vi "五子棋_電腦對戰.vi"() -> ()   [LabVIEW 2019, in "五子棋.lvlib"]
uses:
  Status.ctl
  SetPiece.ctl
  <vilib>/numeric/Random Number (Range) U64.vi
  <vilib>/numeric/sub_Random U32.vi
panel:
  out "Info":string
  out "狀態":string
  out "黑子":T1[][](array[typedef])
  out "白子":T2[][](array[typedef])
  # "五子棋電腦對戰版"
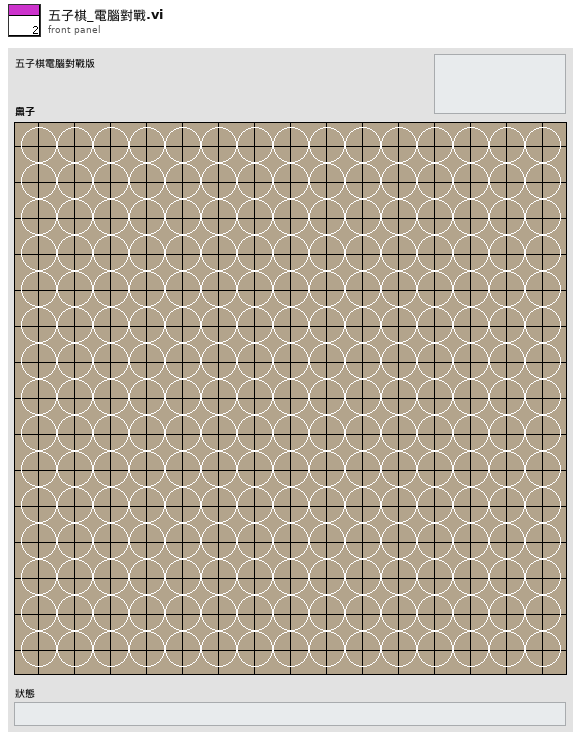
[diagram p1: front panel]
types:
  T1 = typedef "五子棋.lvlib/黑子.ctl" = bool
  T2 = typedef "五子棋.lvlib/白子.ctl" = bool
  T3 = typedef "五子棋.lvlib/SetPiece.ctl" = cluster{"Row":i32, "Col":i32, "Black?":bool}
  T4 = typedef "五子棋.lvlib/Status.ctl" = enum16{"Idle", "Initialize", "Set Piece", "Check Win", "Computer Play"}
  T5 = typedef "LVPositionTypeDef.ctl" = cluster{"Left":i32, "Top":i32}
  T6 = typedef "LVBoundsTypeDef.ctl" = cluster{"Width":u32, "Height":u32}
  T7 = cluster{"Number of Columns":u32, "Number of Rows":u32}
  T8 = typedef "Event 2-上課練習.lvlib/黑子.ctl" = bool
  T9 = typedef "Event 2-上課練習.lvlib/白子.ctl" = bool
  T10 = cluster{"Number of Columns":bool, "Number of Rows":bool}
  T11 = typedef "LVPoint32TypeDef.ctl" = cluster{"Horizontal":i32, "Vertical":i32}
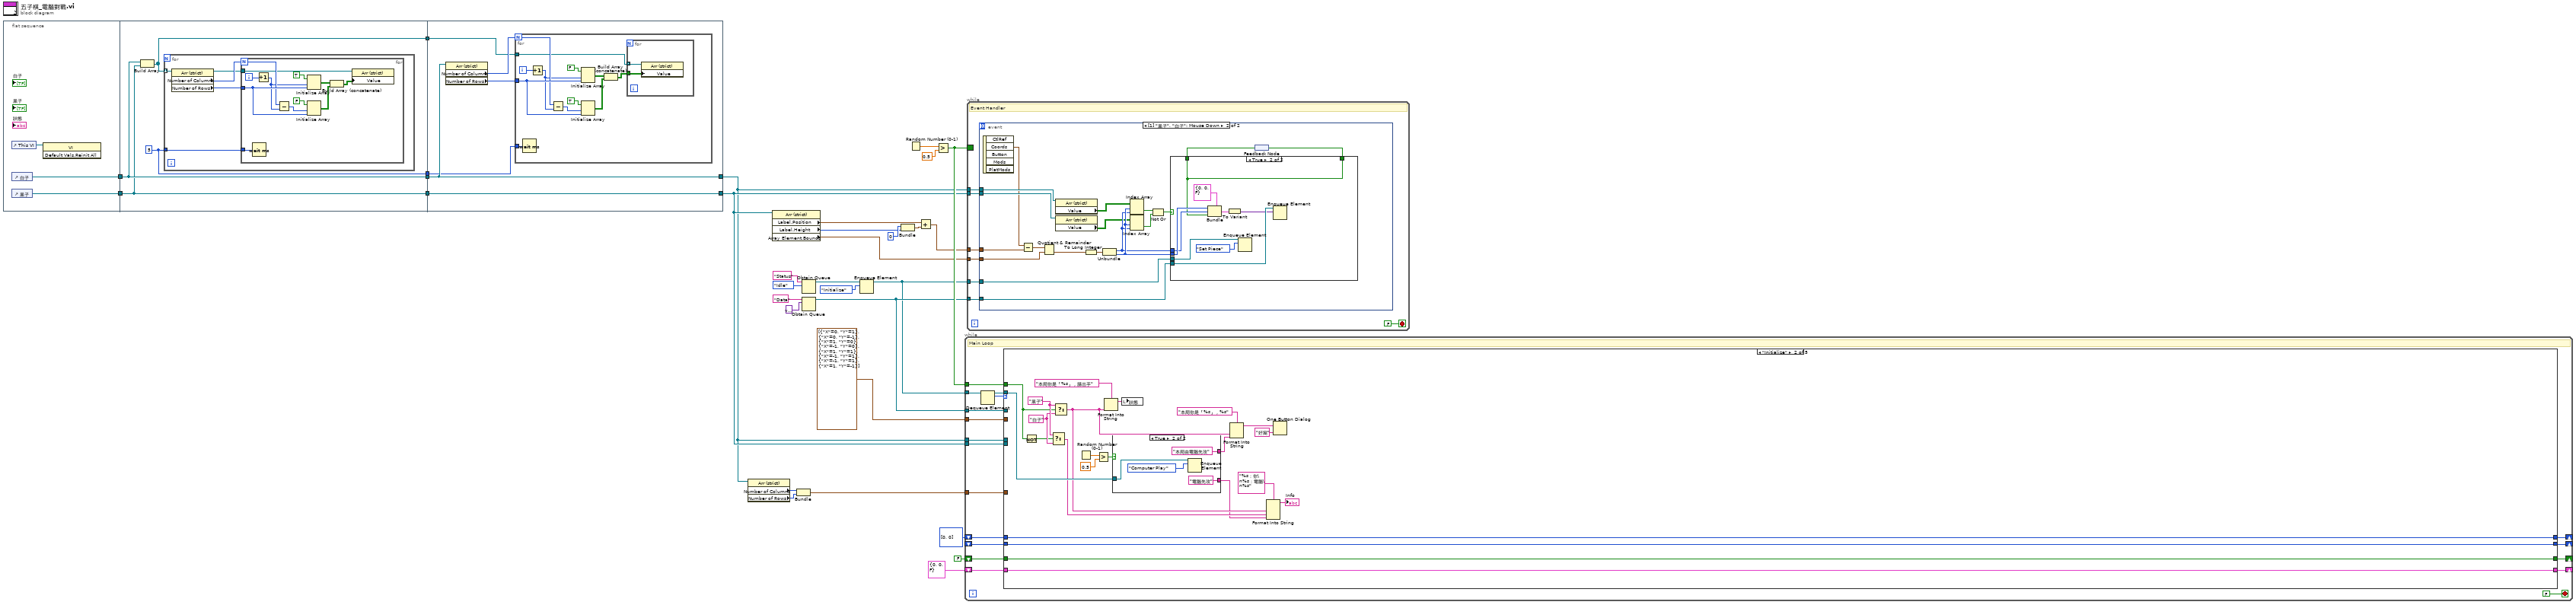
[diagram p0: block diagram]
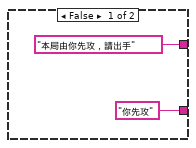
[diagram p3: hidden frame]
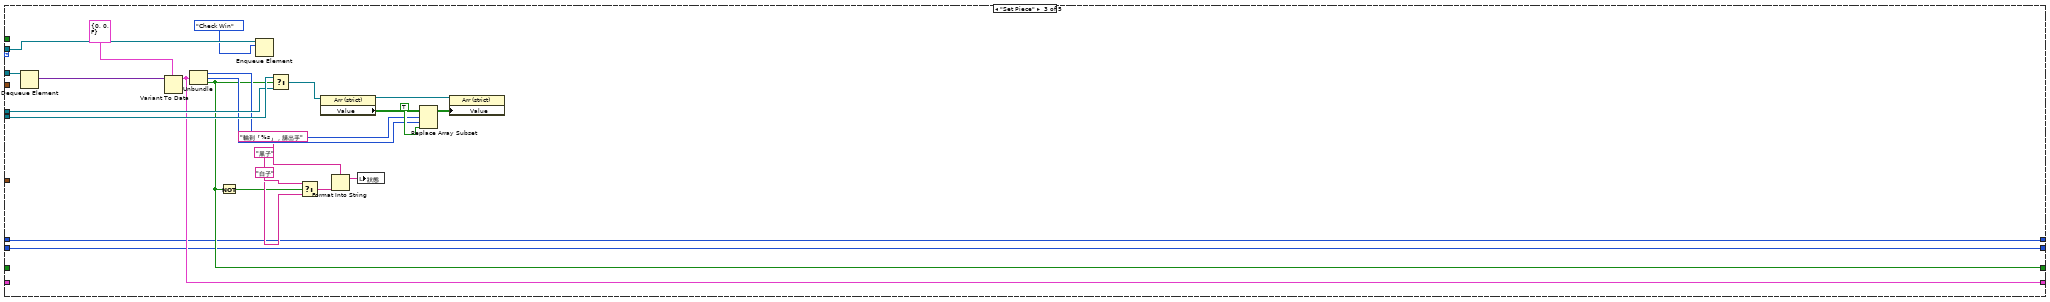
[diagram p4: hidden frame]
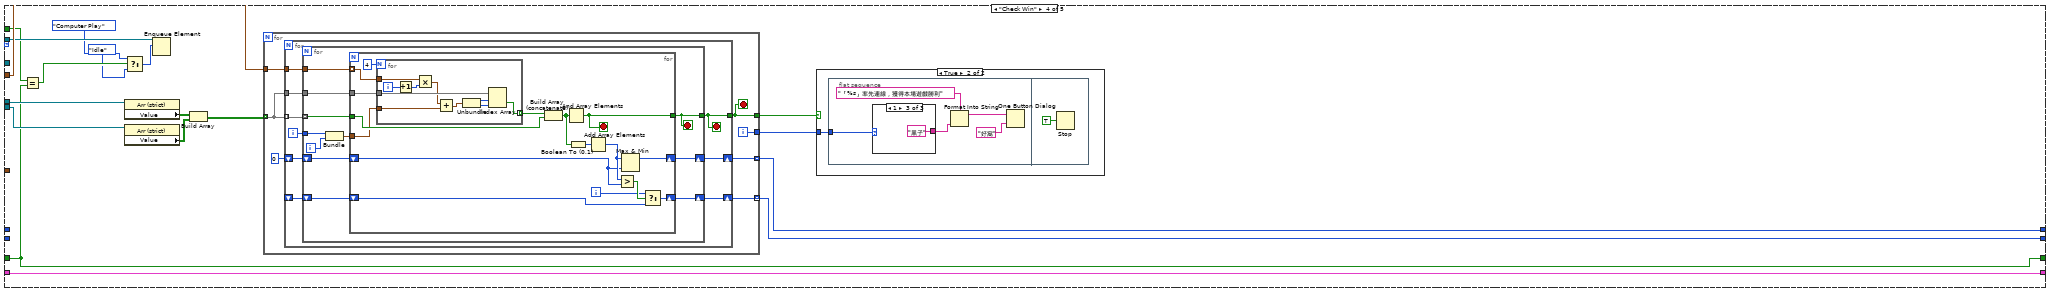
[diagram p5: hidden frame]
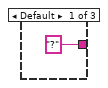
[diagram p7: hidden frame]
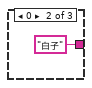
[diagram p8: hidden frame]
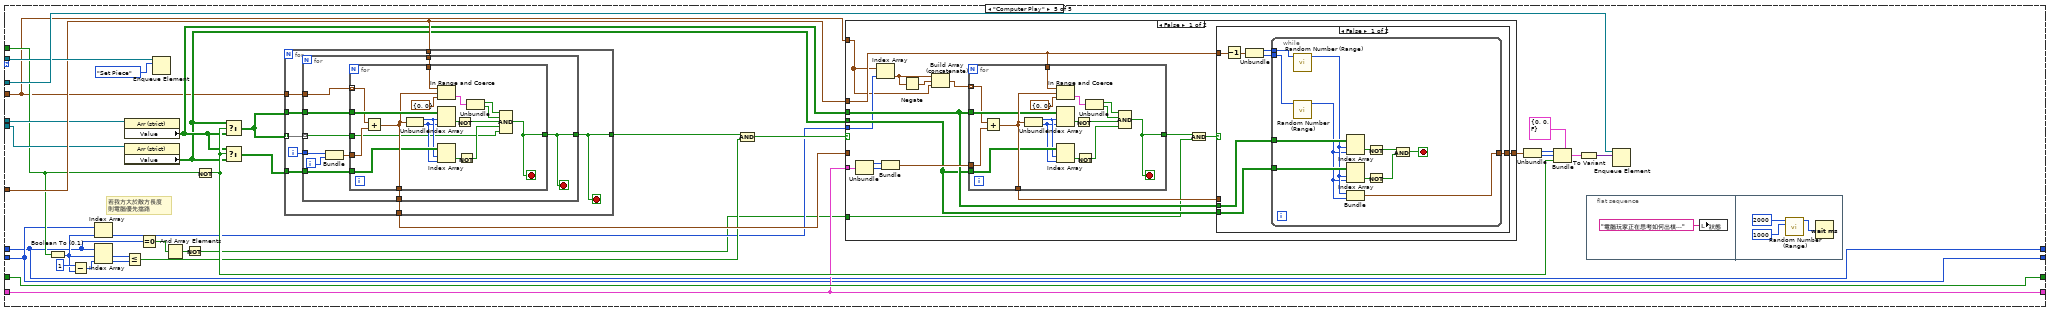
[diagram p9: hidden frame]
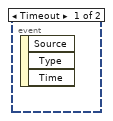
[diagram p12: hidden frame]
diagram:
  n1 = flat-sequence {
    tunnel: [w34] -> w15
    tunnel: [w33] -> w14
    tunnel: w15 -> [w38]
    tunnel: w14 -> [w39]
    tunnel: [w38] -> w13
    tunnel: [w39] -> w12
    tunnel: [w37] -> w11
    tunnel: [w36] -> w1
    tunnel: [w59] -> w8
    tunnel: [w62] -> w26
    tunnel: w13 -> [w62]
    tunnel: w12 -> [w59]
    tunnel: w11 -> [w58]
    tunnel: w1 -> [w57]
    frame #0 {
      n2 = control-ref of="This VI"() -> (w35:refnum<vi>)
      n3 = control-ref of="白子"() -> (w33:refnum<vi>)
      n4 = control-ref of="黑子"() -> (w34:refnum<vi>)
      n5 = invoke class="VI" method="Default Vals.Reinit All"(reference=w35) -> ()  [unwired: 2 in, 3 out]
    }
    frame #1 {
      w36 = u32 5 ("milliseconds to wait")
      n6 = Build Array(w39, w38) -> (w37:refnum<vi>[])
      n7 = for {
        tunnel: w37 -> [w44] mode=indexing
        tunnel: w36 -> [w40]
        n8 = property class="Arr (strict)"(reference=w44) -> (reference out=w41:refnum<vi>, "Number of Columns"=w43:u32, "Number of Rows"=w42:u32)  [unwired: 1 in, 1 out]
        n9 = for {
          N: w43 -> [w52]
          tunnel: w42 -> [w53]
          tunnel: w41 -> [w47]
          tunnel: w40 -> [w45]
          i -> [w55]
          n10 = Wait (ms)(milliseconds to wait=w45) -> ()  [unwired: 1 out]
          n11 = Increment(x=w55) -> (x+1=w51:i32)
          n12 = Subtract(x=w52, y=w51) -> (x-y=w50:i32)
          n13 = Initialize Array(TRUE, w51, w53) -> (w49:bool[][])
          n14 = Initialize Array(FALSE, w50, w53) -> (w48:bool[][])
          n15 = Build Array (concatenate)(w49, w48) -> (w46:bool[][])
          n16 = property class="Arr (strict)"(reference=w47, "Value"=w46) -> ()  [unwired: 1 in, 2 out]
        }
      }
    }
    frame #2 {
      n17 = property class="Arr (strict)"(reference=w59) -> ("Number of Columns"=w61:u32, "Number of Rows"=w60:u32)  [unwired: 1 in, 2 out]
      n18 = for {
        N: w61 -> [w70]
        tunnel: w60 -> [w71]
        tunnel: w58 -> [w64]
        tunnel: w57 -> [w63]
        i -> [w73]
        n19 = Wait (ms)(milliseconds to wait=w63) -> ()  [unwired: 1 out]
        n20 = Increment(x=w73) -> (x+1=w69:i32)
        n21 = Subtract(x=w70, y=w69) -> (x-y=w68:i32)
        n22 = Initialize Array(FALSE, w69, w71) -> (w67:bool[][])
        n23 = Initialize Array(TRUE, w68, w71) -> (w66:bool[][])
        n24 = Build Array (concatenate)(w67, w66) -> (w65:bool[][])
        n25 = for {
          tunnel: w64 -> [w76] mode=indexing
          tunnel: w65 -> [w75]
          n26 = property class="Arr (strict)"(reference=w76, "Value"=w75) -> ()  [unwired: 1 in, 2 out]
        }
      }
    }
  }
  n27 = property class="Arr (strict)"(reference=w8) -> ("Number of Columns"=w7:u32, "Number of Rows"=w6:u32)  [unwired: 1 in, 2 out]
  n28 = property class="Arr (strict)"(reference=w26) -> ("Label.Position"=w25:T5, "Label.Height"=w21:u32, "Array Element.Bounds"=w20:T6)  [unwired: 1 in, 2 out]
  n29 = Bundle("Number of Columns"=w7, "Number of Rows"=w6) -> (w5:T7)  [unwired: 1 in]
  n30 = Obtain Queue(name (unnamed)="Status", element data type=Status."Idle" ("Status")) -> (queue out=w17:refnum<queue>)  [unwired: 3 in, 2 out]
  n31 = Obtain Queue(name (unnamed)="Data", element data type=variant) -> (queue out=w27:refnum<queue>)  [unwired: 3 in, 2 out]
  n32 = Enqueue Element(queue=w17, element=Status."Initialize" ("Status")) -> (queue out=w2:refnum<queue>)  [unwired: 2 in, 2 out]
  n33 = Bundle(0, "Label.Height"=w21) -> (w24:cluster{i32, "Label.Height":u32})  [unwired: 1 in]
  n34 = Random Number (0-1)() -> (number: 0 to 1=w19:dbl)
  n35 = Add(x=w25, y=w24) -> (x+y=w23:cluster{i32, u32})
  n36 = Greater?(x=w19, y=0.5) -> (0:w32:bool)
  n37 = while {
    tunnel: w2 -> [w94]
    tunnel: w27 -> [w88]
    tunnel: w26 -> [w92]
    tunnel: w8 -> [w91]
    tunnel: w32 -> [w87]
    shift-right: [w86] -> _
    shift-left: FALSE ("Black?") -> [w85]
    shift-right: [w84] -> _
    shift-left: T3 {"Row"=0, "Col"=0, "Black?"=FALSE} -> [w83]
    tunnel: w5 -> [w82]
    shift-right: [w81] -> _
    shift-left: i16[] [0, 0] -> [w80]
    shift-right: [w79] -> _
    shift-left: _ -> [w78]
    tunnel: cluster{"X":i32, "Y":i32}[] [{"X"=0, "Y"=1}, {"X"=0, "Y"=-1}, {"X"=1, "Y"=0}, {"X"=-1, "Y"=0}, {"X"=1, "Y"=1}, {"X"=-1, "Y"=1}, {"X"=-1, "Y"=1}, {"X"=1, "Y"=-1}] -> [w77]
    stop <- FALSE stop-if-true
    # "Main Loop"
    n38 = Dequeue Element(queue=w94) -> (queue out=w89:refnum<queue>, element=w93:T4)  [unwired: 2 in, 2 out]
    n39 = case shown="\"Initialize\"" w93 {
      tunnel: w92 -> [_ _ w145 w166 w249]
      tunnel: w91 -> [_ _ w144 w167 w250]
      tunnel: w89 -> [_ w115 w141 w168 w267]
      tunnel: w88 -> [_ _ w139 _ w268]
      tunnel: w87 -> [_ w103 _ w160 w248]
      tunnel: [w98 w119 w131 w159 w266] -> w86
      tunnel: w85 -> [w98 w119 _ w159 w266]
      tunnel: [w97 w118 w130 w154 w251] -> w84
      tunnel: w83 -> [w97 w118 _ w154 w251]
      tunnel: w82 -> [_ _ _ _ w254]
      tunnel: [w96 w117 w129 w153 w236] -> w81
      tunnel: w80 -> [w96 w117 w129 _ w236]
      tunnel: [w95 w116 w128 w152 w241] -> w79
      tunnel: w78 -> [w95 w116 w128 _ w241]
      tunnel: w77 -> [_ _ _ w169 w238]
      frame "Idle", Default {
      }
      frame "Initialize" {
        w104 = "白子"
        w105 = "黑子"
        n40 = Not(x=w103) -> (.not. x?=w102:bool)
        n41 = Select(t=w105, s=w102, f=w104) -> (s? t:f=w101:string)
        n42 = Select(t=w105, s=w103, f=w104) -> (s? t:f=w106:string)
        n43 = Random Number (0-1)() -> (number: 0 to 1=w113:dbl)
        n44 = Greater?(x=w113, y=0.5) -> (0:w111:bool)
        n45 = Format Into String(format string="本局你是「%s」，請出手", w106) -> (resulting string=w120:string)  [unwired: 2 in, 1 out]
        n46 = case shown="True" w111 {
          tunnel: w115 -> [_ w125]
          tunnel: ["本局由你先攻，請出手" ("format string") "本局由電腦先攻" ("format string")] -> w110
          tunnel: ["你先攻" ("format string") "電腦先攻" ("format string")] -> w100
          frame False {
          }
          frame True {
            n47 = Enqueue Element(queue=w125, element=Status."Computer Play" ("Status")) -> ()  [unwired: 2 in, 3 out]
          }
        }
        n48 = local write "狀態"(w120) -> ()
        n49 = Format Into String(format string="本局你是「%s」，%s", w106, w110) -> (resulting string=w109:string)  [unwired: 2 in, 1 out]
        n50 = Format Into String(format string="%s：你\n%s：電腦\n%s", w106, w101, w100) -> (resulting string=→"Info":string)  [unwired: 2 in, 1 out]
        n51 = One Button Dialog(message=w109, button name ("OK")="好窩") -> ()  [unwired: 1 out]
      }
      frame "Set Piece" {
        n52 = Dequeue Element(queue=w139) -> (element=w138:variant)  [unwired: 2 in, 3 out]
        n53 = Variant To Data(type=T3 {"Row"=0, "Col"=0, "Black?"=FALSE}, Variant=w138) -> (data=w130:T3)  [unwired: 1 in, 1 out]
        n54 = Unbundle(w130) -> ("Row"=w143:i32, "Col"=w142:i32, "Black?"=w131:bool)
        n55 = Not(x=w131) -> (.not. x?=w133:bool)
        n56 = Enqueue Element(queue=w141, element=Status."Check Win") -> ()  [unwired: 2 in, 3 out]
        n57 = Select(t=w145, s=w131, f=w144) -> (s? t:f=w148:refnum<vi>)
        n58 = Select(t="黑子", s=w133, f="白子") -> (s? t:f=w134:string)
        n59 = property class="Arr (strict)"(reference=w148) -> (reference out=w146:refnum<vi>, "Value"=w147:T8[][])  [unwired: 1 in, 1 out]
        n60 = Format Into String(format string="輪到「%s」，請出手", w134) -> (resulting string=w132:string)  [unwired: 2 in, 1 out]
        n61 = local write "狀態"(w132) -> ()
        n62 = Replace Array Subset(array=w147, new element=T1 TRUE ("new element/subarray"), index (row)=w143, index (col)=w142) -> (w149:T8[][])
        n63 = property class="Arr (strict)"(reference=w146, "Value"=w149) -> ()  [unwired: 1 in, 2 out]
      }
      frame "Check Win" {
        n64 = Equal?(x=w160, y=w159) -> (x = y?=w158:bool)
        n65 = property class="Arr (strict)"(reference=w167) -> ("Value"=w165:T9[][])  [unwired: 1 in, 2 out]
        n66 = property class="Arr (strict)"(reference=w166) -> ("Value"=w164:T9[][])  [unwired: 1 in, 2 out]
        n67 = Select(t=Status."Computer Play" ("element"), s=w158, f=Status."Idle" ("element")) -> (s? t:f=w157:T4)
        n68 = Enqueue Element(queue=w168, element=w157) -> ()  [unwired: 2 in, 3 out]
        n69 = Build Array(w165, w164) -> (w163:T9[][][])
        n70 = for {
          tunnel: w163 -> [w175] mode=indexing
          tunnel: w169 -> [w176]
          tunnel: [w174] -> w162
          tunnel: [w173] -> w161
          tunnel: [w171] -> w153 mode=indexing
          tunnel: [w170] -> w152 mode=indexing
          i -> [w173]
          stop <- w174 stop-if-true
          n71 = for {
            tunnel: w175 -> [w184] mode=indexing
            tunnel: w176 -> [w185]
            tunnel: w175 -> [w183]
            tunnel: [w182] -> w174
            shift-right: [w180] -> w171
            shift-left: i16 0 -> [w179]
            shift-right: [w178] -> w170
            shift-left: _ -> [w177]
            i -> [w181]
            stop <- w182 stop-if-true
            n72 = for {
              tunnel: w184 -> [w196] mode=indexing
              tunnel: w185 -> [w195]
              tunnel: w183 -> [w194]
              tunnel: [w193] -> w182
              tunnel: w181 -> [w192]
              shift-right: [w189] -> w180
              shift-left: w179 -> [w188]
              shift-right: [w187] -> w178
              shift-left: w177 -> [w186]
              i -> [w191]
              stop <- w193 stop-if-true
              n73 = Bundle(w192, w191) -> (w190:cluster{i32, i32})  [unwired: 1 in]
              n74 = for {
                tunnel: w196 -> [w209]
                tunnel: w195 -> [w207] mode=indexing
                tunnel: w194 -> [w212]
                tunnel: [w208] -> w193
                tunnel: w190 -> [w203]
                shift-right: [w204] -> w189
                shift-left: w188 -> [w201]
                shift-right: [w199] -> w187
                shift-left: w186 -> [w198]
                i -> [w197]
                stop <- w208 stop-if-true
                n75 = for {
                  N: 4 -> [_]
                  tunnel: w212 -> [w222]
                  tunnel: [w219] -> w210 mode=indexing
                  tunnel: w203 -> [w218]
                  tunnel: w207 -> [w216]
                  i -> [w217]
                  n76 = Increment(x=w217) -> (x+1=w215:i32)
                  n77 = Multiply(x=w216, y=w215) -> (x*y=w214:cluster{"X":i32, "Y":i32})
                  n78 = Add(x=w214, y=w218) -> (x+y=w213:cluster{i32, i32})
                  n79 = Unbundle(w213) -> (w221:i32, w220:i32)
                  n80 = Index Array(array=w222, index (row)=w221, index (col)=w220) -> (element=w219:T9)
                }
                n81 = Build Array (concatenate)(w210, w209) -> (w206:T9[])
                n82 = And Array Elements(Boolean array=w206) -> (logical AND=w208:bool)
                n83 = Boolean To (0,1)(Boolean=w206) -> (0, 1=w205:i16[])
                n84 = Add Array Elements(numeric array=w205) -> (sum=w202:i16)
                n85 = Greater?(x=w202, y=w201) -> (0:w200:bool)
                n86 = Max & Min(x=w202, y=w201) -> (max(x,y)=w204:i16)  [unwired: 1 out]
                n87 = Select(t=w197, s=w200, f=w198) -> (s? t:f=w199:i32)
              }
            }
          }
        }
        n88 = case shown="True" w162 {
          tunnel: w161 -> [_ w223]
          frame False {
          }
          frame True {
            n89 = flat-sequence {
              tunnel: w223 -> [w227]
              frame #0 {
                n90 = case shown="1" w227 {
                  tunnel: ["?" "白子" "黑子"] -> w226
                  frame Default {
                  }
                  frame 0 {
                  }
                  frame 1 {
                  }
                }
                n91 = Format Into String(format string="「%s」率先連線，獲得本場遊戲勝利", w226) -> (resulting string=w225:string)  [unwired: 2 in, 1 out]
                n92 = One Button Dialog(message=w225, button name ("OK")="好窩") -> ()  [unwired: 1 out]
              }
              frame #1 {
                n93 = Stop(stop? (T)=TRUE) -> ()
              }
            }
          }
        }
      }
      frame "Computer Play" {
        # "若我方大於敵方長度\n則電腦優先擋路"
        n94 = Boolean To (0,1)(Boolean=w248) -> (0, 1=w240:i16)
        n95 = Subtract(x=i16 1, y=w240) -> (x-y=w246:i16)
        n96 = Index Array(array=w241, index=w240) -> (element=w239:i32)
        n97 = Index Array(array=w236, index #1=w240, index #2=w246) -> (element #1=w245:i16, element #2=w237:i16)
        n98 = property class="Arr (strict)"(reference=w250) -> ("Value"=w253:T9[][])  [unwired: 1 in, 2 out]
        n99 = property class="Arr (strict)"(reference=w249) -> ("Value"=w252:T9[][])  [unwired: 1 in, 2 out]
        n100 = Less Or Equal?(x=w245, y=w237) -> (x <= y?=w242:bool)
        n101 = Equal To 0?(x=w236) -> (x = 0?=w235:bool[])
        n102 = Enqueue Element(queue=w267, element=Status."Set Piece") -> ()  [unwired: 2 in, 3 out]
        n103 = And Array Elements(Boolean array=w235) -> (logical AND=w234:bool)
        n104 = Not(x=w234) -> (.not. x?=w233:bool)
        n105 = Not(x=w248) -> (.not. x?=w263:bool)
        n106 = Select(t=w252, s=w263, f=w253) -> (s? t:f=w264:T9[][])
        n107 = Select(t=w253, s=w263, f=w252) -> (s? t:f=w262:T9[][])
        n108 = for {
          tunnel: w264 -> [w335] mode=indexing
          tunnel: w264 -> [w334]
          tunnel: [w333] -> w244
          tunnel: [w331] -> w255
          tunnel: w262 -> [w330]
          tunnel: w254 -> [w329]
          tunnel: w238 -> [w328]
          i -> [w332]
          stop <- w333 stop-if-true
          n109 = for {
            tunnel: w335 -> [w345] mode=indexing
            tunnel: w334 -> [w344]
            tunnel: [w343] -> w333
            tunnel: w332 -> [w342]
            tunnel: [w339] -> w331
            tunnel: w330 -> [w338]
            tunnel: w329 -> [w337]
            tunnel: w328 -> [w336]
            i -> [w341]
            stop <- w343 stop-if-true
            n110 = Bundle(w342, w341) -> (w340:cluster{i32, i32})  [unwired: 1 in]
            n111 = for {
              tunnel: w345 -> [w347]
              tunnel: w336 -> [w346] mode=indexing
              tunnel: w344 -> [w363]
              tunnel: [w361] -> w343
              tunnel: w340 -> [w362]
              tunnel: [w360] -> w339
              tunnel: w338 -> [w359]
              tunnel: w337 -> [w358]
              stop <- w361 stop-if-true
              n112 = Add(x=w346, y=w362) -> (x+y=w360:cluster{i32, i32})
              n113 = Unbundle(w360) -> (w356:i32, w355:i32)
              n114 = Index Array(array=w363, index (row)=w356, index (col)=w355) -> (element=w357:T9)
              n115 = Index Array(array=w359, index (row)=w356, index (col)=w355) -> (element=w354:T9)
              n116 = In Range and Coerce(upper limit=w358, x=w360, lower limit=T7 {"Number of Columns"=0, "Number of Rows"=0}) -> (In Range?=w350:T10)  [unwired: 1 out]
              n117 = Not(x=w357) -> (.not. x?=w353:T9)
              n118 = Not(x=w354) -> (.not. x?=w352:T9)
              n119 = Unbundle(w350) -> ("Number of Columns"=w348:bool, "Number of Rows"=w349:bool)
              n120 = Compound Arithmetic op=AND(w348, w349, w353, w352, w347) -> (w361:T9)
            }
          }
        }
        n121 = Compound Arithmetic op=AND(w244, w242) -> (w243:T9)
        n122 = case shown="False" w243 {
          tunnel: [w285 w327] -> w256
          tunnel: w255 -> [_ w327]
          tunnel: w254 -> [w283 _]
          tunnel: w253 -> [w282 _]
          tunnel: w252 -> [w281 _]
          tunnel: w251 -> [w289 _]
          tunnel: w238 -> [w277 _]
          tunnel: w239 -> [w280 _]
          tunnel: w233 -> [w273 _]
          frame False {
            n123 = Unbundle(w289) -> ("Row"=w288:i32, "Col"=w287:i32)  [unwired: 1 out]
            n124 = Index Array(array=w277, index=w280) -> (element=w279:cluster{"X":i32, "Y":i32})
            n125 = Bundle("Row"=w288, "Col"=w287) -> (w286:cluster{"Row":i32, "Col":i32})  [unwired: 1 in]
            n126 = Negate(x=w279) -> (-x=w278:cluster{"X":i32, "Y":i32})
            n127 = Build Array (concatenate)(w279, w278, w277) -> (w276:cluster{"X":i32, "Y":i32}[])
            n128 = for {
              tunnel: w282 -> [w311]
              tunnel: [w325] -> w275
              tunnel: w286 -> [w326]
              tunnel: [w324] -> w284
              tunnel: w281 -> [w323]
              tunnel: w283 -> [w322]
              tunnel: w276 -> [w310] mode=indexing
              stop <- w325 stop-if-true
              n129 = Add(x=w310, y=w326) -> (x+y=w324:cluster{i32, i32})
              n130 = Unbundle(w324) -> (w320:i32, w319:i32)
              n131 = Index Array(array=w311, index (row)=w320, index (col)=w319) -> (element=w321:T9)
              n132 = Index Array(array=w323, index (row)=w320, index (col)=w319) -> (element=w318:T9)
              n133 = In Range and Coerce(upper limit=w322, x=w324, lower limit=T7 {"Number of Columns"=0, "Number of Rows"=0}) -> (In Range?=w314:T10)  [unwired: 1 out]
              n134 = Not(x=w321) -> (.not. x?=w317:T9)
              n135 = Not(x=w318) -> (.not. x?=w316:T9)
              n136 = Unbundle(w314) -> ("Number of Columns"=w312:bool, "Number of Rows"=w313:bool)
              n137 = Compound Arithmetic op=AND(w312, w313, w317, w316) -> (w325:T9)
            }
            n138 = And(x=w275, y=w273) -> (x .and. y?=w274:T9)
            n139 = case shown="False" w274 {
              tunnel: [w292 w309] -> w285
              tunnel: w284 -> [_ w309]
              tunnel: w283 -> [w291 _]
              tunnel: w282 -> [w294 _]
              tunnel: w281 -> [w293 _]
              frame False {
                n140 = Decrement(x=w291) -> (x-1=w290:T7)
                n141 = Unbundle(w290) -> ("Number of Columns"=w296:u32, "Number of Rows"=w295:u32)
                n142 = while {
                  tunnel: w296 -> [w308]
                  tunnel: w295 -> [w307]
                  tunnel: w294 -> [w306]
                  tunnel: w293 -> [w305]
                  tunnel: [w297] -> w292
                  stop <- w300 stop-if-true
                  n143 = call-poly <vilib>:"Random Number (Range).vi"("upper bound (100)"=w308) -> ("number"=w299:u64)  [unwired: 10 in]
                  n144 = call-poly <vilib>:"Random Number (Range).vi"("upper bound (100)"=w307) -> ("number"=w298:u64)  [unwired: 10 in]
                  n145 = Bundle("number"=w299, "number"=w298) -> (w297:cluster{"number":u64, "number":u64})  [unwired: 1 in]
                  n146 = Index Array(array=w306, index (row)=w299, index (col)=w298) -> (element=w304:T9)
                  n147 = Index Array(array=w305, index (row)=w299, index (col)=w298) -> (element=w303:T9)
                  n148 = Not(x=w304) -> (.not. x?=w302:T9)
                  n149 = Not(x=w303) -> (.not. x?=w301:T9)
                  n150 = And(x=w302, y=w301) -> (x .and. y?=w300:T9)
                }
              }
              frame True {
              }
            }
          }
          frame True {
          }
        }
        n151 = Unbundle(w256) -> ("number"=w258:u64, "number"=w257:u64)
        n152 = Bundle(cluster=T3 {"Row"=0, "Col"=0, "Black?"=FALSE}, "Row"=w258, "Col"=w257, "Black?"=w263) -> (w260:T3)
        n153 = To Variant(anything=w260) -> (Variant=w261:variant)
        n154 = flat-sequence {
          frame #0 {
            n155 = local write "狀態"("電腦玩家正在思考如何出棋..." ("狀態")) -> ()
          }
          frame #1 {
            n156 = call-poly <vilib>:"Random Number (Range).vi"("lower bound (0)"=u64 1000, "upper bound (100)"=u64 2000 ("lower bound (0)")) -> ("number"=w270:u64)  [unwired: 9 in]
            n157 = Wait (ms)(milliseconds to wait=w270) -> ()  [unwired: 1 out]
          }
        }
        n158 = Enqueue Element(queue=w268, element=w261) -> ()  [unwired: 2 in, 3 out]
      }
    }
  }
  n159 = while {
    tunnel: w26 -> [w369]
    tunnel: w8 -> [w368]
    tunnel: w20 -> [w367]
    tunnel: w2 -> [w366]
    tunnel: w27 -> [w365]
    tunnel: w23 -> [w364]
    border: w32 -> [_]
    stop <- FALSE stop-if-true
    # "Event Handler"
    n160 = event shown="[1] \"黑子\", \"白子\": Mouse Down" {
      selector: _ -> [_ _]
      dyn-events: _ -> [_ _]
      timeout: _ -> [_ _]
      tunnel: w369 -> [_ w387]
      tunnel: w368 -> [_ w388]
      tunnel: w367 -> [_ w374]
      tunnel: w366 -> [_ w379]
      tunnel: w365 -> [_ w378]
      tunnel: w364 -> [_ w376]
      event Timeout {
        n161 = event-data() -> ()  [unwired: 1 in, 3 out]
      }
      event "黑子", "白子": Mouse Down {
        n162 = event-data() -> ("Coords"=w377:T11)  [unwired: 1 in, 4 out]
        n163 = Subtract(x=w377, y=w376) -> (x-y=w375:cluster{i32, u32})
        n164 = Quotient & Remainder(x=w375, y=w374) -> (floor(x/y)=w373:T6)  [unwired: 1 out]
        n165 = property class="Arr (strict)"(reference=w388) -> ("Value"=w386:T8[][])  [unwired: 1 in, 2 out]
        n166 = property class="Arr (strict)"(reference=w387) -> ("Value"=w383:T8[][])  [unwired: 1 in, 2 out]
        n167 = To Long Integer(number=w373) -> (32bit integer=w389:cluster{"Width":i32, "Height":i32})
        n168 = Unbundle(w389) -> ("Width"=w384:i32, "Height"=w385:i32)
        n169 = Index Array(array=w386, index (row)=w385, index (col)=w384) -> (element=w382:T8)
        n170 = Index Array(array=w383, index (row)=w385, index (col)=w384) -> (element=w381:T8)
        n171 = Not Or(1:w381, 2:w382) -> (0:w380:T8)
        n172 = feedback #1() -> (w371:bool)
        n173 = case shown="True" w380 {
          tunnel: w385 -> [_ w396]
          tunnel: w384 -> [_ w395]
          tunnel: w379 -> [_ w399]
          tunnel: w378 -> [_ w394]
          tunnel: [w390 w391] -> w372
          tunnel: w371 -> [w390 w391]
          frame False {
          }
          frame True {
            n174 = Bundle(cluster=T3 {"Row"=0, "Col"=0, "Black?"=FALSE}, "Row"=w396, "Col"=w395, "Black?"=w391) -> (w393:T3)
            n175 = To Variant(anything=w393) -> (Variant=w392:variant)
            n176 = Enqueue Element(queue=w399, element=Status."Set Piece") -> ()  [unwired: 2 in, 3 out]
            n177 = Enqueue Element(queue=w394, element=w392) -> ()  [unwired: 2 in, 3 out]
          }
        }
        n178 = feedback-in #1(w372) -> ()
      }
    }
  }
